vi "CryoCon Get Calib Info.vi"(0 "VISA session":refnum<visa-resource-name>, 1 "Index":i32) -> (4 "dup VISA session":refnum<visa-resource-name>, 5 "Sensor Name":string, 6 "Sensor Type 2":T1=enum."DC Resistance 625 ½", 7 "Multiplier":dbl)   [LabVIEW 2024]
uses:
  Sub Controls/CryoCon Sensor Type.ctl
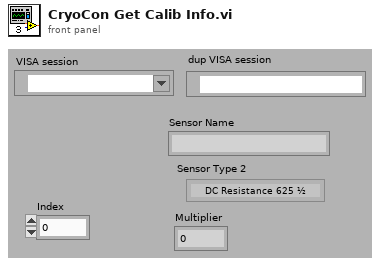
[diagram p1: front panel]
types:
  T1 = typedef "CryoCon Sensor Type.ctl" = enum16{"Diode", "AC Resistance", "DC Resistance 3.1 k½", "DC Resistance 312 ½", "DC Resistance 625 ½"}
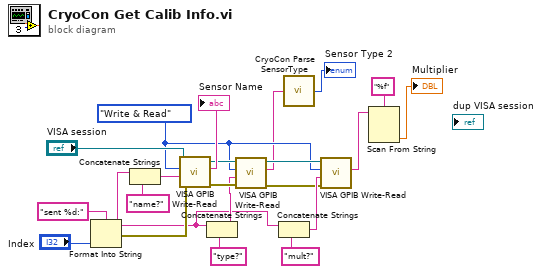
[diagram p0: block diagram]
diagram:
  w8 = enum16{"Write", "Read", "Write & Read"}."Write & Read" ("Action")
  n1 = Format Into String(format string="sent %d:" ("Format String"), "Index") -> (resulting string=w7:string, error out=w14:errorcluster)  [unwired: 2 in]
  n2 = Concatenate Strings(w7, "name?" ("string")) -> (w16:string)
  n3 = call "VISA GPIB Write-Read.vi"("error in (no error)"=w14, "Command"=w16, "Action"=w8, "VISA resource name"="VISA session") -> ("error out"=w17:errorcluster, "String Returned"=→"Sensor Name":string, "dup VISA Session"=w18:refnum<visa-resource-name>)  [unwired: 4 in, 1 out]
  n4 = Concatenate Strings(w7, "type?" ("string")) -> (w12:string)
  n5 = call "VISA GPIB Write-Read.vi"("error in (no error)"=w17, "Command"=w12, "Action"=w8, "VISA resource name"=w18) -> ("error out"=w6:errorcluster, "String Returned"=w2:string, "dup VISA Session"=w11:refnum<visa-resource-name>)  [unwired: 4 in, 1 out]
  n6 = Concatenate Strings(w7, "mult?" ("string")) -> (w9:string)
  n7 = call "CryoCon Parse SensorType.vi"("String Read"=w2) -> ("Sensor Type 2"=→"Sensor Type 2":T1)
  n8 = call "VISA GPIB Write-Read.vi"("error in (no error)"=w6, "Command"=w9, "Action"=w8, "VISA resource name"=w11) -> ("String Returned"=w5:string)  [unwired: 4 in, 3 out]
  n9 = Scan From String(format string="%f", input string=w5) -> (output 1=→"Multiplier":dbl)  [unwired: 3 in, 3 out]
